vi "Get NT Class.vi"(8 "error in (no error)":errorcluster, 11 "PV Data in":refnum<class "PV Data.lvclass">) -> (0 "error out":errorcluster, 2 "NT Base out":refnum<class "NT Base.lvclass">, 3 "PV Data out":refnum<class "PV Data.lvclass">)   [LabVIEW 2020, in "PV Access.lvlib" / "PV Data.lvlib" / "PV Data.lvclass"]
uses:
  PV Data.lvclass
  NT Base/NT Base.lvclass
  NT Scalar/NT Scalar.lvclass
  NT Scalar (Numeric)/NT Scalar (Numeric).lvclass
  <vilib>/ErrorRing/Error Ring.xnode
  PV Data.lvclass/PV Data.ctl
  C:/Users/eyw68381/source/repos/pvaccess-labview/labview/source/PV Data/NT Base/NT Base.lvclass
  C:/Users/eyw68381/source/repos/pvaccess-labview/labview/source/PV Data/NT Scalar/NT Scalar.lvclass
  C:/Users/eyw68381/source/repos/pvaccess-labview/labview/source/PV Data/NT Scalar (Numeric)/NT Scalar (Numeric).lvclass
  NT Enum/NT Enum.lvclass
  C:/Users/eyw68381/source/repos/pvaccess-labview/labview/source/PV Data/NT Enum/NT Enum.lvclass
  PV Data.lvlib
  <vilib>/Utility/error.llb/Error Cluster From Error Code.vi
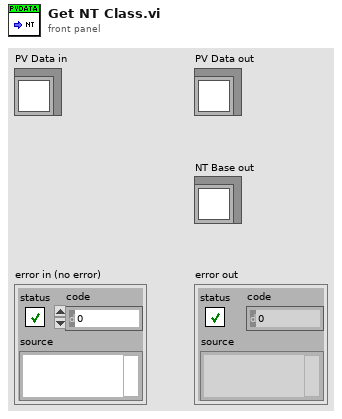
[diagram p1: front panel]
types:
  T1 = typedef "PV Access.lvlib/PV Data.lvlib/Type Code.ctl" = enum8{"Null", "Bool", "BoolA", "Int8", "Int8A", "Int16", "Int16A", "Int32", "Int32A", "Int64", "Int64A", "UInt8", "UInt8A", "UInt16", "UInt16A", "UInt32", "UInt32A", "UInt64", "UInt64A", "Float32", "Float32A", "Float64", "Float64A", "String", "StringA", "Struct", "StructA", "Union", "UnionA", "Any", "AnyA"}
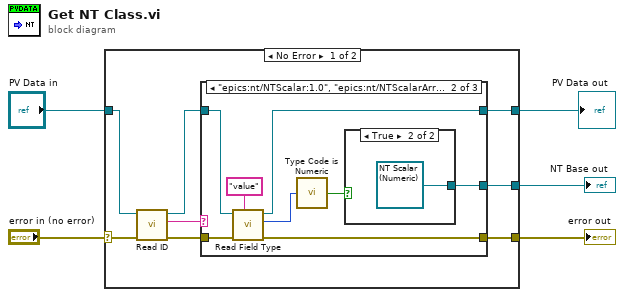
[diagram p0: block diagram]
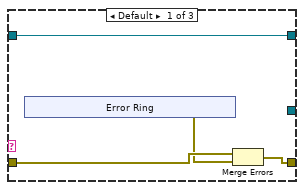
[diagram p2: hidden frame]
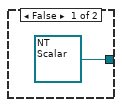
[diagram p3: hidden frame]
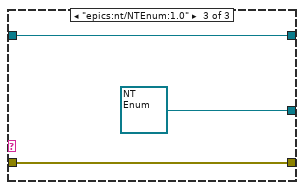
[diagram p4: hidden frame]
diagram:
  n1 = case shown="No Error" "error in (no error)" {
    selector: "error in (no error)" -> [w13 w36]
    tunnel: [w7 w36] -> w1
    tunnel: "PV Data in" -> [w12 w35]
    tunnel: [w8 w35] -> w4
    tunnel: [w6 _] -> w3
    frame No Error {
      n2 = call "Read ID.vi"("error in (no error)"=w13, "PV Data in"=w12) -> ("error out"=w9:errorcluster, "ID"=w11:string, "PV Data out"=w10:refnum<class "PV Data.lvclass">)  [unwired: 7 in]
      n3 = case shown="\"epics:nt/NTScalar:1.0\", \"epics:nt/NTScalarArray:1.0\"" w11 {
        tunnel: w10 -> [w17 w28 w34]
        tunnel: [w15 w22 w32] -> w7
        tunnel: w9 -> [w16 w29 w32]
        tunnel: [_ w24 refnum<class "NT Enum.lvclass"> refnum ("Value.lvlib:NT Scalar (Numeric).lvclass")] -> w6
        tunnel: [w17 w23 w34] -> w8
        frame Default {
          n4 = xnode "Error Ring"() -> ("error out"=w14:errorcluster)
          n5 = Merge Errors(w16, w14) -> (w15:errorcluster)
        }
        frame "epics:nt/NTScalar:1.0", "epics:nt/NTScalarArray:1.0" {
          n6 = call "Read Field Type.vi"("field name"="value", "error in (no error)"=w29, "PV Data in"=w28) -> ("error out"=w22:errorcluster, "type code"=w26:T1, "PV Data out"=w23:refnum<class "PV Data.lvclass">)  [unwired: 6 in]
          n7 = call "Type Code is Numeric.vi"("type code"=w26) -> ("is match?"=w25:bool)
          n8 = case shown="True" w25 {
            tunnel: [refnum<class "NT Scalar.lvclass"> refnum ("Value.lvlib:NT Scalar.lvclass") refnum<class "NT Scalar (Numeric).lvclass"> refnum ("Value.lvlib:NT Scalar (Numeric).lvclass")] -> w24
            frame False {
            }
            frame True {
            }
          }
        }
        frame "epics:nt/NTEnum:1.0" {
        }
      }
    }
    frame Error {
    }
  }
  "error out" <- w1
  "PV Data out" <- w4
  "NT Base out" <- w3
